vi "DAQ_Dyn Dig Gen Configure and Generate.vi"(0 "DAQmx Task In":refnum<k21>, 5 "Timing & Trigger Settings":T1={"Timing Settings"={"Sample Clock Source"="OnboardClock", "Sample Rate (Hz)"=10000.0, "Active Edge"=10280}, "Trigger Settings"={"Trigger Type"=enum."No Trigger", "Digital Start Trigger Source"="", "Digital Start Trigger Edge"=10280}} {"Trigger Settings"."Digital Start Trigger Edge" items=["Rising"=10280, "Falling"=10171]; "Timing Settings"."Active Edge" items=["Rising"=10280, "Falling"=10171]; "Timing Settings"."Sample Rate (Hz)" format="%.2p"}, 7 "Port Digital Data":u32[](array[numeric]), 11 "error in":errorcluster) -> (4 "DAQmx Task Out":refnum<k21>, 6 "Generation Time (s)":dbl format="%.2p", 15 "error out":errorcluster)   [LabVIEW 2021, in "DAQ_Dynamic Digital Pattern Generation.lvlib"]
doc: "Configure, initiate and generate dynamic digital patterns in the channels configured."
uses:
  DAQ_Dynamic Digital Pattern Generation.lvlib
  Typedefs/Timing & Trigger Settings.ctl
  Typedefs/Timing Settings.ctl
  Typedefs/Trigger Settings.ctl
  <vilib>/DAQmx/write.llb/DAQmx Write (Digital 2D U32 NChan NSamp).vi
  <vilib>/DAQmx/configure/timing.llb/DAQmx Timing (Sample Clock).vi
  <vilib>/DAQmx/configure/trigger.llb/DAQmx Start Trigger (Digital Edge).vi
  <vilib>/DAQmx/miscellaneous.llb/DAQmx Fill In Error Info.vi
  <resource>/objmgr/daqmx.rc
panel:
  # "Inputs"
  # "Outputs"
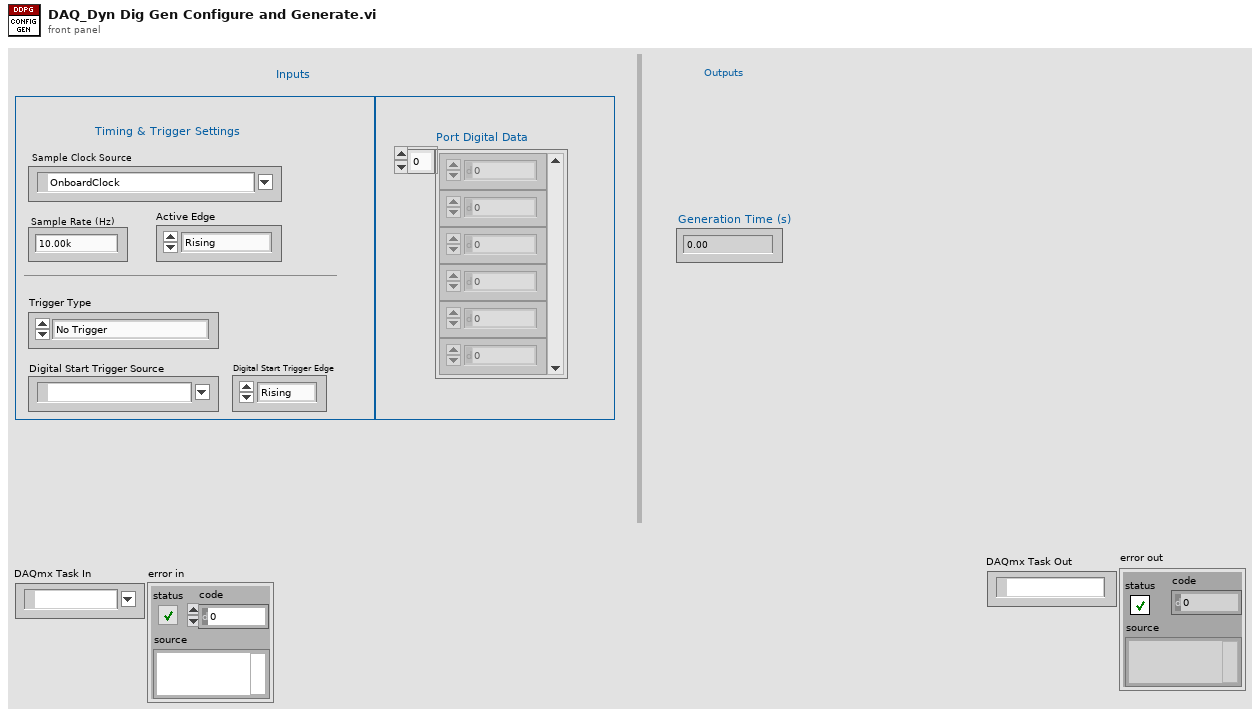
[diagram p1: front panel]
types:
  T1 = typedef "DAQ_Dynamic Digital Pattern Generation.lvlib/Timing & Trigger Settings.ctl" = cluster{"Timing Settings":T2, "Trigger Settings":T3}
  T2 = typedef "DAQ_Dynamic Digital Pattern Generation.lvlib/Timing Settings.ctl" = cluster{"Sample Clock Source":tag, "Sample Rate (Hz)":dbl, "Active Edge":i32}
  T3 = typedef "DAQ_Dynamic Digital Pattern Generation.lvlib/Trigger Settings.ctl" = cluster{"Trigger Type":enum16{"No Trigger", "Digital Start"}, "Digital Start Trigger Source":tag, "Digital Start Trigger Edge":i32}
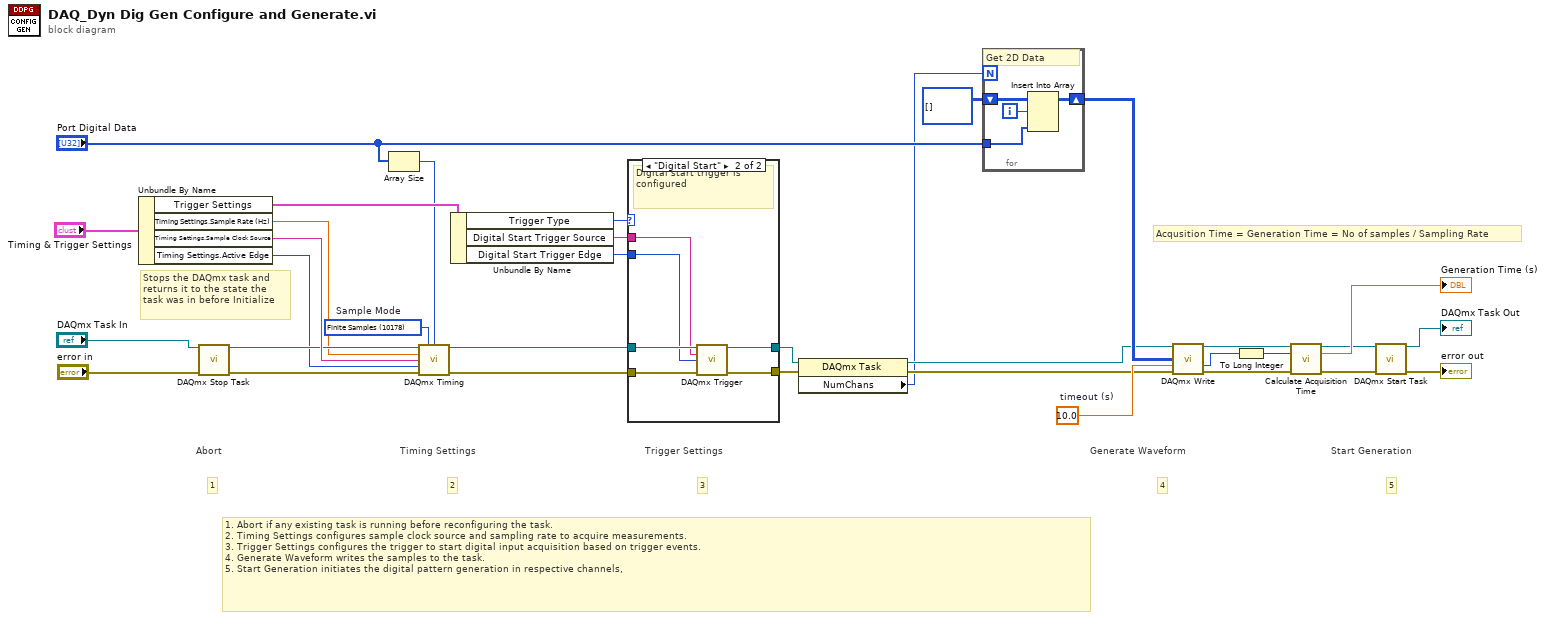
[diagram p0: block diagram]
diagram:
  w23 = 10.0  # timeout (s)
  w24 = 10178 items=["Finite Samples"=10178, "Continuous Samples"=10123, "Hardware Timed Single Point"=12522]  # Sample Mode
  # "Acqusition Time = Generation Time = No of samples / Sampling Rate"
  # "4"
  # "Generate Waveform"
  # "Stops the DAQmx task and returns it to the state the task was in before Initialize"
  # "5"
  # "Start Generation"
  # "1"
  # "Abort"
  # "3"
  # "2"
  # "Trigger Settings"
  # "Timing Settings"
  # "1. Abort if any existing task is running before reconfiguring the task.\n2. Timing Settings configures sample clock source and sampling rate to acquire measurements.\n3. Trigger Settings configures the trigger to start digital input acquisition based on trigger events.\n4. Generate Waveform writes the samples to the task.\n5. Start Generation initiates the digital pattern generation in respective channels,"
  n1 = Unbundle By Name("Timing & Trigger Settings") -> ("Trigger Settings"=w27:T3, "Timing Settings.Sample Rate (Hz)"=w11:dbl, "Timing Settings.Sample Clock Source"=w32:tag, "Timing Settings.Active Edge"=w2:i32)
  n2 = call <vilib>:"DAQmx Stop Task.vi"("task/channels in"="DAQmx Task In", "error in"="error in") -> ("task out"=w25:refnum<k21>, "error out"=w26:errorcluster)  [unwired: 12 in]
  n3 = Array Size(array="Port Digital Data") -> (size(s)=w12:i32)
  n4 = call-poly <vilib>:"DAQmx Timing.vi"("task/channels in"=w25, "sample mode"=w24, "samples per channel"=w12, "rate"=w11, "source"=w32, "active edge"=w2, "error in"=w26) -> ("task out"=w19:refnum<k21>, "error out"=w20:errorcluster)  [unwired: 7 in]
  n5 = Unbundle By Name(w27) -> ("Trigger Type"=w28:enum16{"No Trigger", "Digital Start"}, "Digital Start Trigger Source"=w30:tag, "Digital Start Trigger Edge"=w29:i32)
  n6 = case shown="\"Digital Start\"" w28 {
    tunnel: w19 -> [w36 w42]
    tunnel: w20 -> [w35 w41]
    tunnel: [w36 w40] -> w7
    tunnel: [w35 w39] -> w6
    tunnel: w30 -> [_ w38]
    tunnel: w29 -> [_ w37]
    frame Default {
      # "No Trigger settings has been configured"
    }
    frame "Digital Start" {
      # "Digital start trigger is configured"
      n7 = call-poly <vilib>:"DAQmx Trigger.vi"("task/channels in"=w42, "source"=w38, "edge"=w37, "error in"=w41) -> ("task out"=w40:refnum<k21>, "error out"=w39:errorcluster)  [unwired: 10 in]
    }
  }
  n8 = property class="DAQmx Task"(reference=w7, error in=w6) -> (reference out=w4:refnum<k21>, error out=w5:errorcluster, "NumChans"=w3:u32)
  n9 = for {
    N: w3 -> [_]
    shift-right: [w45] -> w8
    shift-left: u32[][] [] -> [w46]
    tunnel: "Port Digital Data" -> [w44]
    i -> [w43]
    # "Get 2D Data"
    n10 = Insert Into Array(array=w46, index (row)=w43, new element=w44) -> (w45:u32[][])  [unwired: 1 in]
  }
  n11 = call-poly <vilib>:"DAQmx Write.vi"("task/channels in"=w4, "data"=w8, "timeout"=w23, "error in"=w5) -> ("task out"=w17:refnum<k21>, "number of samples written per channel"=w14:u32, "error out"=w16:errorcluster)  [unwired: 9 in]
  n12 = To Long Integer(number=w14) -> (32bit integer=w13:i32)
  n13 = call "Calculate Acquisition Time.vi"("Refnum in"=w17, "Number of Samples"=w13, "error in (no error)"=w16) -> ("Refnum out"=w18:refnum<k21>, "Acquisition Time Period (s)"=→"Generation Time (s)":dbl, "error out"=w15:errorcluster)  [unwired: 10 in]
  n14 = call <vilib>:"DAQmx Start Task.vi"("task/channels in"=w18, "error in"=w15) -> ("task out"=→"DAQmx Task Out":refnum<k21>, "error out"=→"error out":errorcluster)  [unwired: 12 in]
